vi "Process Pupil Reflection_ovalROI2.vi"(0 "Image In":T2, 3 "Threshold":u8=130, 4 "Direction to keep":enum16{"Above", "Below"}(ring)=enum."Below", 5 "error in (no error)":errorcluster, 6 "Display":bool, 7 "Fit type":enum16{"Circle", "Ellipse"}(ring)=enum."Ellipse", 8 "Global Rectangle":i32[](array[numeric]), 9 "Subsampling":i32=1, 10 "Color":u32(colorbox)=16711680, 11 "use % thresh":bool, 12 "Display Overlay":bool, 13 "Points to show":enum16{"All points", "Fit points"}(ring)) -> (14 "Image out":T2, 15 "x position":dbl, 17 "y position":dbl, 18 "diameter":dbl, 19 "error out":errorcluster)   [LabVIEW 2013]
uses:
  <vilib>/vision/Image Controls.llb/IMAQ Image.ctl
  Outline/Outline.lvclass
  <vilib>/Analysis/baseanly.llb/Mean (DBL).vi
  <vilib>/vision/NI_Vision_Development_Module.lvlib
  <vilib>/Analysis/NI_AALBase.lvlib
panel:
  in  "ID":enum32{"External", "Internal"}(ring)
  in  "Type":u32=4
  in  "ROI Descriptor":T1 {"Contours"."Type" items=["No Selection", "Point", "Line", "Rectangle", "Oval", "Polygon", "Freehand Region", "Annulus", "Unused2", "Unused3", "Broken Line", "Freehand Line", "Rotated Rectangle"]}
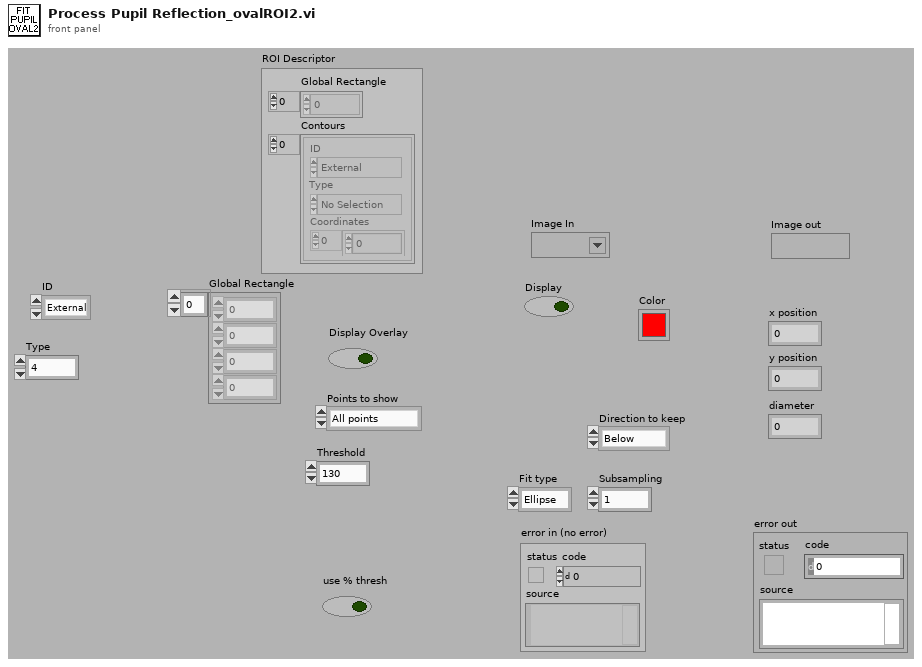
[diagram p1: front panel]
types:
  T1 = typedef "ROI Descriptor" = cluster{"Global Rectangle":i32[], "Contours":cluster{"ID":enum32{"External", "Internal"}, "Type":u32, "Coordinates":i32[]}[]}
  T2 = typedef "IMAQ Image.ctl" = refnum<image>
  T3 = cluster{"ID":enum32{"External", "Internal"}, "Type":u32, "Global Rectangle":i32[]}
  T4 = cluster{"ID":enum32{"External", "Internal"}, "Type":u32, "Global Rectangle":i32[]}[]
  T5 = cluster{"Center":cluster{"X":sgl, "Y":sgl}, "Radius":dbl}
  T6 = cluster{"Center":cluster{"X":sgl, "Y":sgl}, "Major Axis":cluster{"Point 1":cluster{"X":sgl, "Y":sgl}, "Point 2":cluster{"X":sgl, "Y":sgl}}, "Minor Axis":cluster{"Point 1":cluster{"X":sgl, "Y":sgl}, "Point 2":cluster{"X":sgl, "Y":sgl}}}
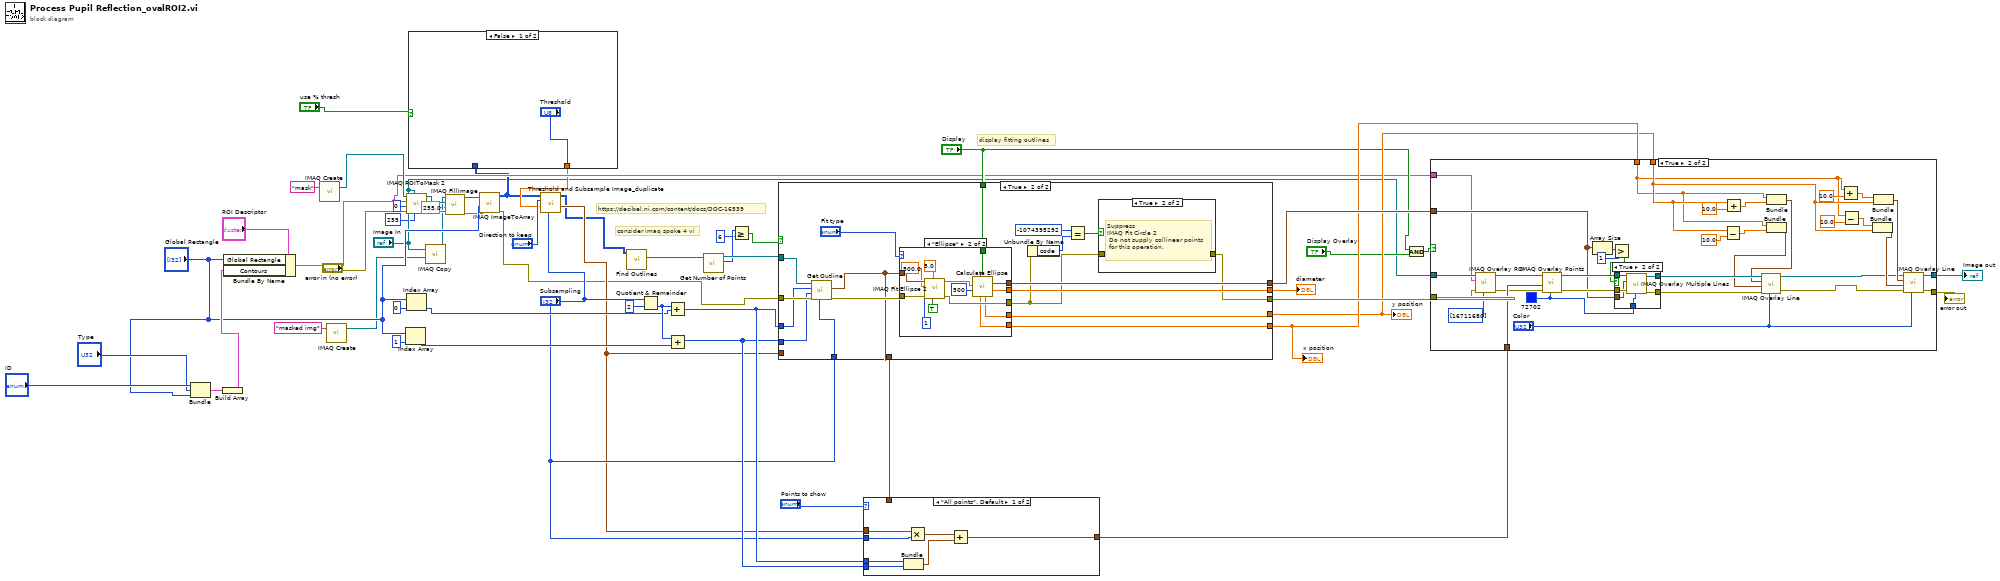
[diagram p0: block diagram]
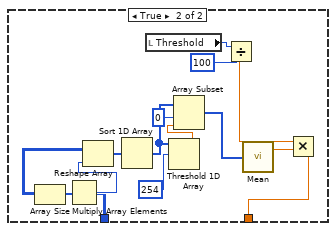
[diagram p2: hidden frame]
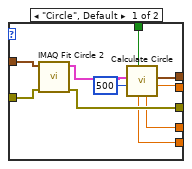
[diagram p8: hidden frame]
diagram:
  # "https://decibel.ni.com/content/docs/DOC-16539"
  # "consider imaq spoke 4 vi"
  # "display fitting outlines"
  n1 = Bundle("ID"="ID", "Type"="Type", "Global Rectangle"="Global Rectangle") -> (w21:T3)  [unwired: 1 in]
  n2 = Build Array(w21) -> (w18:T4)
  n3 = Bundle By Name(cluster="ROI Descriptor", "Global Rectangle"="Global Rectangle", "Contours"=w18) -> (w22:T1)
  n4 = call "IMAQ Create"("Image Name"="mask") -> ("New Image"=w27:T2)  [unwired: 4 in, 1 out]
  n5 = call "IMAQ Create"("Image Name"="masked img") -> ("New Image"=w6:T2)  [unwired: 4 in, 1 out]
  n6 = Index Array(array="Global Rectangle", index=1) -> (element=w50:i32)
  n7 = call "IMAQ ROIToMask 2"("Background Value (0)"=255, "Image Model"="Image In", "error in (no error)"="error in (no error)", "Filling Value (255)"=0, "ROI Descriptor"=w22, "Image"=w27) -> ("error out"=w10:errorcluster, "Image Out"=w8:T2)  [unwired: 3 in, 1 out]
  n8 = Index Array(array="Global Rectangle", index=0) -> (element=w53:i32)
  n9 = call "IMAQ Copy"("Image Dst"=w6, "Image Src"="Image In") -> ("Image Dst Out"=w4:T2)  [unwired: 4 in, 1 out]
  n10 = call "IMAQ FillImage"("error in (no error)"=w10, "Pixel Value (U8, U16, I16, Float)"=sgl 255.0, "Image Mask"=w8, "Image"=w4) -> ("error out"=w9:errorcluster, "Image Out"=w7:T2)  [unwired: 6 in]
  n11 = call "IMAQ ImageToArray"("error in (no error)"=w9, "Optional Rectangle"="Global Rectangle", "Image"=w7) -> ("error out"=w11:errorcluster, "Image Pixels (U8)"=w14:u8[][])  [unwired: 1 in, 3 out]
  n12 = case shown="False" "use % thresh" {
    tunnel: w14 -> [_ w68]
    tunnel: ["Threshold" w66] -> w15
    frame False {
    }
    frame True {
      n13 = Array Size(array=w68) -> (size(s)=w69:i32[])
      n14 = Multiply Array Elements(1:w69) -> (0:w70:i32)
      n15 = Reshape Array(w68, w70) -> (w62:u8[])
      n16 = Sort 1D Array(array=w62) -> (sorted array=w60:u8[])
      n17 = local read "Threshold"() -> (w65:u8)
      n18 = Threshold 1D Array(2:i16 254 ("threshold y"), 3:w60) -> (0:w59:dbl)  [unwired: 1 in]
      n19 = Array Subset(array=w60, index=0, length=w59) -> (w57:u8[])
      n20 = Divide(x=w65, y=u8 100) -> (x/y=w64:dbl)
      n21 = call-poly <vilib>:"Mean.vi"("X"=w57) -> ("mean"=w67:dbl)  [unwired: 1 out]
      n22 = Multiply(x=w64, y=w67) -> (x*y=w66:dbl)
    }
  }
  n23 = call "Threshold and Subsample Image_duplicate.vi"("Subsample"="Subsampling", "Threshold"=w15, "Direction to keep"="Direction to keep", "Image Pixels (U8)"=w14) -> ("Cross Threshold Points"=w13:cluster{"X":i32, "Y":i32}[], "Image Pixels (U8) out"=w12:u8[][])  [unwired: 6 in]
  n24 = call "Find Outlines.vi"("Image Pixels (U8)"=w12) -> ("Largest Outline"=w45:refnum<class "Outline.lvclass">)  [unwired: 9 in, 1 out]
  n25 = Quotient & Remainder(x="Subsampling", y=2) -> (floor(x/y)=w54:i32)  [unwired: 1 out]
  n26 = Add(x=w54, y=w53) -> (x+y=w35:i32)
  n27 = Add(x=w54, y=w50) -> (x+y=w34:i32)
  n28 = call-dynamic "Get Number of Points.vi"("Outline in"=w45) -> ("Number of points"=w48:i32, "Outline out"=w49:refnum<class "Outline.lvclass">)  [unwired: 8 in, 1 out]
  n29 = Greater Or Equal?(x=w48, y=6) -> (x >= y?=w46:bool)
  n30 = case shown="True" w46 {
    tunnel: w11 -> [w71 w89]
    tunnel: [w71 w77] -> w44
    tunnel: w35 -> [_ w74]
    tunnel: w34 -> [_ w73]
    tunnel: w49 -> [_ w88]
    tunnel: "Subsampling" -> [_ w75]
    tunnel: [_ w86] -> w43
    tunnel: [_ w84] -> w42
    tunnel: [_ w83] -> w41
    tunnel: [_ w82] -> w38
    tunnel: "Display" -> [_ w76]
    tunnel: w13 -> [_ _]
    tunnel: [_ w72] -> w37
    frame False {
    }
    frame True {
      n31 = call-dynamic "Get Outline.vi"("Scale Factor"=w75, "error in (no error)"=w89, "Y Offset"=w73, "X Offset"=w74, "Outline in"=w88) -> ("error out"=w85:errorcluster, "Outline"=w72:cluster{"X":i32, "Y":i32}[])  [unwired: 4 in, 1 out]
      n32 = case shown="\"Ellipse\"" "Fit type" {
        tunnel: w85 -> [w99 w114]
        tunnel: w72 -> [w100 w113]
        tunnel: [w98 w112] -> w78
        tunnel: [w96 w110] -> w86
        tunnel: [w95 w105] -> w84
        tunnel: [w94 w104] -> w83
        tunnel: [w92 w102] -> w82
        tunnel: w76 -> [w91 w101]
        frame "Circle", Default {
          n33 = call "IMAQ Fit Circle 2"("error in (no error)"=w99, "Radial Points"=w100) -> ("error out"=w98:errorcluster, "Circle"=w97:T5)  [unwired: 4 in, 4 out]
          n34 = call "Calculate Circle.vi"("Display"=w91, "steps"=500, "Circle"=w97) -> ("Diameter"=w92:dbl, "Circle Coordinates"=w96:cluster{"X":i32, "Y":i32}[], "y position"=w94:dbl, "x position"=w95:dbl)  [unwired: 5 in]
        }
        frame "Ellipse" {
          n35 = call "IMAQ Fit Ellipse 2"("Reject Outliers (FALSE)"=TRUE, "Pixel Radius"=5.0, "error in (no error)"=w114, "Maximum Iterations"=1, "Minimum Score"=500.0, "Radial Points"=w113) -> ("error out"=w112:errorcluster, "Ellipse"=w109:T6)  [unwired: 4 out]
          n36 = call "Calculate Ellipse.vi"("Display"=w101, "steps"=500, "Ellipse"=w109) -> ("Effective Diameter"=w102:sgl, "Ellipse Coordinates"=w110:cluster{"X":i32, "Y":i32}[], "y position"=w104:dbl, "x position"=w105:dbl)  [unwired: 5 in]
        }
      }
      n37 = Unbundle By Name(w78) -> ("code"=w81:i32)
      n38 = Equal?(x=-1074395292, y=w81) -> (x = y?=w79:bool)
      n39 = case shown="True" w79 {
        tunnel: w78 -> [w90 _]
        tunnel: [w90 _] -> w77
        frame False {
        }
        frame True {
          # "Suppress\nIMAQ Fit Circle 2\n Do not supply collinear points\n for this operation."
        }
      }
    }
  }
  "diameter" <- w38
  "x position" <- w42
  "y position" <- w41
  n40 = case shown="\"All points\", Default" "Points to show" {
    tunnel: w13 -> [w119 _]
    tunnel: "Subsampling" -> [w118 _]
    tunnel: w35 -> [w117 _]
    tunnel: w34 -> [w116 _]
    tunnel: [w115 w122] -> w33
    tunnel: w37 -> [_ w122]
    frame "All points", Default {
      n41 = Bundle(w117, w116) -> (w121:cluster{i32, i32})  [unwired: 1 in]
      n42 = Multiply(x=w119, y=w118) -> (x*y=w120:cluster{"X":i32, "Y":i32}[])
      n43 = Add(x=w120, y=w121) -> (x+y=w115:cluster{i32, i32}[])
    }
    frame "Fit points" {
    }
  }
  n44 = And(x="Display", y="Display Overlay") -> (x .and. y?=w30:bool)
  n45 = case shown="True" w30 {
    tunnel: w44 -> [w124 w131]
    tunnel: "Image In" -> [w123 w133]
    tunnel: w43 -> [_ w154]
    tunnel: [w124 w143] -> w40
    tunnel: w42 -> [_ w139]
    tunnel: w41 -> [_ w142]
    tunnel: [w123 w136] -> w39
    tunnel: w33 -> [_ w134]
    tunnel: w22 -> [_ w129]
    frame False {
    }
    frame True {
      w125 = u32 72702 ("Color")
      n46 = call "IMAQ Overlay ROI"("Colors (Green)"=u32[] [16711680], "error in (no error)"=w131, "ROI Descriptor"=w129, "Image"=w133) -> ("error out"=w130:errorcluster, "Image Out"=w132:T2)  [unwired: 6 in]
      n47 = call "IMAQ Overlay Points"("Color"=w125, "error in (no error)"=w130, "Array of Points"=w134, "Image"=w132) -> ("error out"=w158:errorcluster, "Image Out"=w159:T2)  [unwired: 6 in]
      n48 = Array Size(array=w154) -> (size(s)=w157:i32)
      n49 = Greater?(x=w157, y=1) -> (0:w155:bool)
      n50 = case shown="True" w155 {
        tunnel: w159 -> [w161 w167]
        tunnel: w158 -> [w160 w166]
        tunnel: [w161 w165] -> w152
        tunnel: [w160 w164] -> w153
        tunnel: w154 -> [_ w163]
        tunnel: w125 -> [_ w162]
        frame False {
        }
        frame True {
          n51 = call "IMAQ Overlay Multiple Lines"("Color"=w162, "error in (no error)"=w166, "Line End Points"=w163, "Image"=w167) -> ("error out"=w164:errorcluster, "Image Out"=w165:T2)  [unwired: 6 in]
        }
      }
      n52 = Subtract(x=w142, y=10.0) -> (x-y=w147:dbl)
      n53 = Add(x=w142, y=10.0) -> (x+y=w150:dbl)
      n54 = Bundle("x position"=w139, w147) -> (w146:cluster{"x position":dbl, dbl})  [unwired: 1 in]
      n55 = Bundle("x position"=w139, w150) -> (w149:cluster{"x position":dbl, dbl})  [unwired: 1 in]
      n56 = call "IMAQ Overlay Line"("Color"="Color", "error in (no error)"=w153, "End Point"=w146, "Start Point"=w149, "Image"=w152) -> ("error out"=w127:errorcluster, "Image Out"=w126:T2)  [unwired: 5 in]
      n57 = Add(x=w139, y=10.0) -> (x+y=w138:dbl)
      n58 = Subtract(x=w139, y=10.0) -> (x-y=w137:dbl)
      n59 = Bundle(w137, "y position"=w142) -> (w144:cluster{dbl, "y position":dbl})  [unwired: 1 in]
      n60 = Bundle(w138, "y position"=w142) -> (w145:cluster{dbl, "y position":dbl})  [unwired: 1 in]
      n61 = call "IMAQ Overlay Line"("Color"="Color", "error in (no error)"=w127, "End Point"=w144, "Start Point"=w145, "Image"=w126) -> ("error out"=w143:errorcluster, "Image Out"=w136:T2)  [unwired: 5 in]
    }
  }
  "error out" <- w40
  "Image out" <- w39
